vi "move_to_absolute_position_with_feedback.vi"(0 "device_index (in) [0=def]":i32, 5 "Error In":errorcluster) -> (19 "Error Out":errorcluster)   [LabVIEW 2013, in "examples.lvlib"]
doc: "Move the motor at the specified index to an absolute position with realtime feedback about the state of the motor.\n\nProduced By:\n\n<B>Kod Integrations, LLC</B>\n4835 Marianne Drive\nMount Airy, MD 21771\nhttp://www.kodintegrations.com\nemail: info@kodintegrations.com\nphone: (240) 687-1288"
uses:
  libraries/examples.lvlib
  classes/Controller/_Controller.lvclass
  common/controls/motor_enabled_state_axes_group.ctl
  libraries/common.lvlib
  common/controls/motor_status.ctl
  common/controls/axis.ctl
  common/controls/movement_item.ctl
panel:
  out "motion_state":T1=enum."CONST"
  out "response":string
  out "success?":bool
  in  "target_value (in)":i32
  in  "axis (def=X)":T2
  in  "clear_buffer? (T)":bool=TRUE
  # "instructions:\n\nAt the specified device index, enter a target position\nvalue and (for multi-controller applications only) a\nspecific axis and run the VI.  The VI will continue to\nrun until the motor has returned to an IDLE state\n(motion_state).\n\nNOTE: This example VI makes an attempt to enable\nthe motor at the targeted axis.  If left disabled, the\nmove command will appear to be successful, but\nthe motor physically does not respond.\n\nLikewise, once the state has returned to IDLE, the\noutput will be disabled once again."
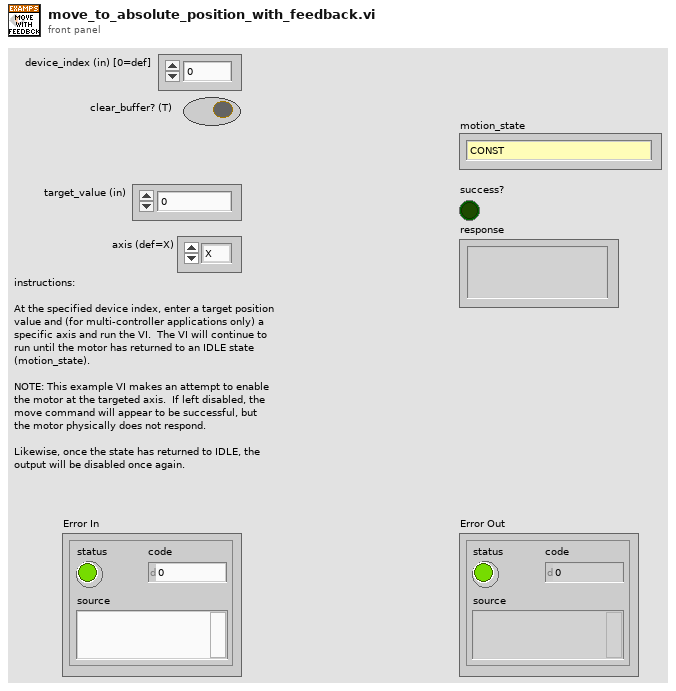
[diagram p1: front panel]
types:
  T1 = typedef "common.lvlib/motor_status.ctl" = enum16{"IDLE", "CONST", "ACCEL", "DECEL", "HOME_SWITCH", "-LIMIT_SWITCH", "+LIMIT_SWITCH", "-LIMIT_ERR", "+LIMIT_ERR", "COMM_TIMEOUT", "ALARM_INPUT", "ALARM_ERROR", "TOC_TIMEOUT_STATUS", "LATCH_INPUT_STATUS", "Z_INDEX_STATUS"}
  T2 = typedef "common.lvlib/axis.ctl" = enum16{"X", "Y", "Z", "U"}
  T3 = typedef "common.lvlib/movement_item.ctl" = cluster{"axis":T2, "target":i32}
  T4 = typedef "common.lvlib/motor_enabled_state_axes_group.ctl" = cluster{"x-axis":bool, "y-axis":bool, "z-axis":bool, "u-axis":bool}
  T5 = typedef "common.lvlib/complete_motor_state.ctl" = cluster{"X":T6, "Y":T6, "Z":T6, "U":T6, "buffer_enabled?":bool, "buffer_start":i32, "buffer_end":i32, "avail_buffer":i32, "move_mode":T7}
  T6 = typedef "common.lvlib/single_axis_state.ctl" = cluster{"motion_state":T1, "other_states":T1[]}
  T7 = typedef "common.lvlib/move_mode.ctl" = enum16{"ABSOLUTE", "INCREMENTAL"}
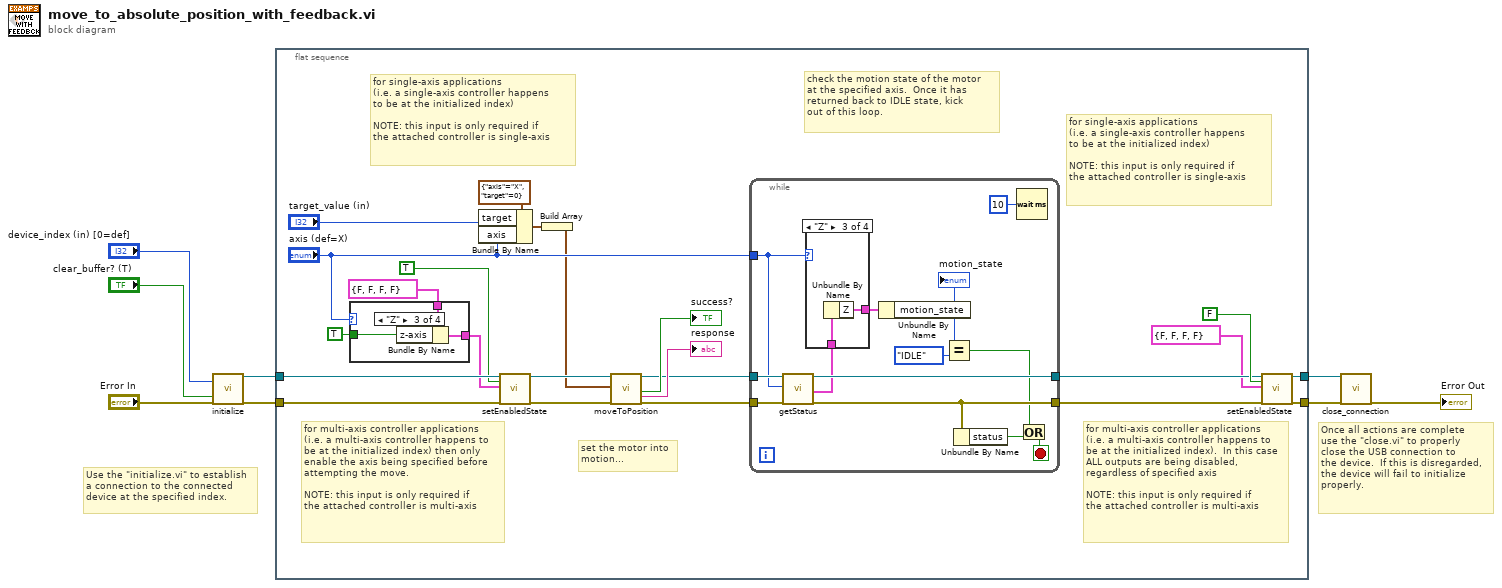
[diagram p0: block diagram]
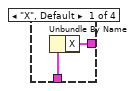
[diagram p2: hidden frame]
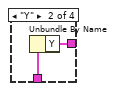
[diagram p3: hidden frame]
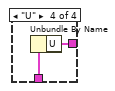
[diagram p4: hidden frame]
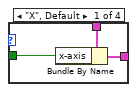
[diagram p5: hidden frame]
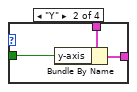
[diagram p6: hidden frame]
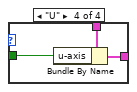
[diagram p7: hidden frame]
diagram:
  # "Once all actions are complete\nuse the \"close.vi\" to properly\nclose the USB connection to \nthe device.  If this is disregarded,\nthe device will fail to initialize \nproperly."
  # "Use the \"initialize.vi\" to establish\na connection to the connected\ndevice at the specified index."
  n1 = call "initialize.vi"("device_index (in) [0=def]"="device_index (in) [0=def]", "clear_buffer? (T)"="clear_buffer? (T)", "error in (no error)"="Error In") -> ("reference (out)"=w5:refnum<class "_Controller.lvclass">, "error out"=w4:errorcluster)  [unwired: 15 in]
  n2 = flat-sequence {
    tunnel: w5 -> [w29]
    tunnel: w4 -> [w28]
    tunnel: [w15] -> w3
    tunnel: [w14] -> w2
    frame #0 {
      # "for multi-axis controller applications\n(i.e. a multi-axis controller happens to\nbe at the initialized index).  In this case\nALL outputs are being disabled,\nregardless of specified axis\n\nNOTE: this input is only required if\nthe attached controller is multi-axis"
      # "for single-axis applications\n(i.e. a single-axis controller happens\nto be at the initialized index)\n\nNOTE: this input is only required if\nthe attached controller is single-axis"
      # "check the motion state of the motor\nat the specified axis.  Once it has\nreturned back to IDLE state, kick\nout of this loop."
      # "set the motor into\nmotion..."
      # "for single-axis applications\n(i.e. a single-axis controller happens\nto be at the initialized index)\n\nNOTE: this input is only required if\nthe attached controller is single-axis"
      # "for multi-axis controller applications\n(i.e. a multi-axis controller happens to\nbe at the initialized index) then only \nenable the axis being specified before\nattempting the move.\n\nNOTE: this input is only required if\nthe attached controller is multi-axis"
      n3 = case shown="\"Z\"" "axis (def=X)" {
        tunnel: T4 {"x-axis"=FALSE, "y-axis"=FALSE, "z-axis"=FALSE, "u-axis"=FALSE} ("axes_states (for multi-axis applications only)") -> [w55 w58 w61 w64]
        tunnel: [w54 w57 w60 w63] -> w23
        tunnel: TRUE -> [w53 w56 w59 w62]
        frame "X", Default {
          n4 = Bundle By Name(cluster=w55, "x-axis"=w53) -> (w54:T4)
        }
        frame "Y" {
          n5 = Bundle By Name(cluster=w58, "y-axis"=w56) -> (w57:T4)
        }
        frame "Z" {
          n6 = Bundle By Name(cluster=w61, "z-axis"=w59) -> (w60:T4)
        }
        frame "U" {
          n7 = Bundle By Name(cluster=w64, "u-axis"=w62) -> (w63:T4)
        }
      }
      n8 = Bundle By Name(cluster=T3 {"axis"=enum."X", "target"=0} ("item"), "target"="target_value (in)", "axis"="axis (def=X)") -> (w10:T3)
      n9 = call-dynamic "setEnabledState.vi"("Controller in"=w29, "state (for single-axis applications only) - (def = DISABLED)"=TRUE ("state (for single-axis applications only)"), "axes_states (for multi-axis applications only) - (def = DISABLED)"=w23, "error in (no error)"=w28) -> ("Controller out"=w27:refnum<class "_Controller.lvclass">, "error out"=w26:errorcluster)  [unwired: 12 in, 2 out]
      n10 = Build Array(w10) -> (w9:T3[])
      n11 = call-dynamic "moveToPosition.vi"("Controller in"=w27, "target(s) (in)"=w9, "error in (no error)"=w26) -> ("Controller out"=w21:refnum<class "_Controller.lvclass">, "success?"=→"success?":bool, "response"=→"response":string, "error out"=w20:errorcluster)  [unwired: 13 in]
      n12 = while {
        tunnel: w21 -> [w44]
        tunnel: w20 -> [w43]
        tunnel: "axis (def=X)" -> [w34]
        tunnel: [w42] -> w18
        tunnel: [w40] -> w17
        stop <- w37 stop-if-true
        n13 = call-dynamic "getStatus.vi"("reference (in)"=w44, "axis (def=X)"=w34, "error in (no error)"=w43) -> ("reference (out)"=w42:refnum<class "_Controller.lvclass">, "full_state"=w35:T5, "error out"=w40:errorcluster)  [unwired: 13 in, 1 out]
        n14 = case shown="\"Z\"" w34 {
          tunnel: w35 -> [w46 w48 w50 w52]
          tunnel: [w45 w47 w49 w51] -> w33
          frame "X", Default {
            n15 = Unbundle By Name(w46) -> ("X"=w45:T6)
          }
          frame "Y" {
            n16 = Unbundle By Name(w48) -> ("Y"=w47:T6)
          }
          frame "Z" {
            n17 = Unbundle By Name(w50) -> ("Z"=w49:T6)
          }
          frame "U" {
            n18 = Unbundle By Name(w52) -> ("U"=w51:T6)
          }
        }
        n19 = Unbundle By Name(w33) -> ("motion_state"=w32:T1)
        "motion_state" <- w32
        n20 = Equal?(x=w32, y=motor_status."IDLE" ("motion_state")) -> (x = y?=w39:bool)
        n21 = Unbundle By Name(w40) -> ("status"=w38:bool)
        n22 = Wait (ms)(milliseconds to wait=u32 10) -> ()  [unwired: 1 out]
        n23 = Or(x=w39, y=w38) -> (x .or. y?=w37:bool)
      }
      n24 = call-dynamic "setEnabledState.vi"("Controller in"=w18, "state (for single-axis applications only) - (def = DISABLED)"=FALSE ("state (for single-axis applications only)"), "axes_states (for multi-axis applications only) - (def = DISABLED)"=T4 {"x-axis"=FALSE, "y-axis"=FALSE, "z-axis"=FALSE, "u-axis"=FALSE} ("axes_states (for multi-axis applications only)"), "error in (no error)"=w17) -> ("Controller out"=w15:refnum<class "_Controller.lvclass">, "error out"=w14:errorcluster)  [unwired: 12 in, 2 out]
    }
  }
  n25 = call "close_connection.vi"("reference (in)"=w3, "error in (no error)"=w2) -> ("error out"=→"Error Out":errorcluster)  [unwired: 16 in, 1 out]
